vi "IDEGlobals.vi"(6 "task":T1(ring)=enum."write pause", 9 "Port":string, 10 "Last Path":path, 11 "pause?":bool) -> (1 "Port out":string, 2 "Last Path out":path, 3 "pause? out":bool)   [LabVIEW 2022 SP3]
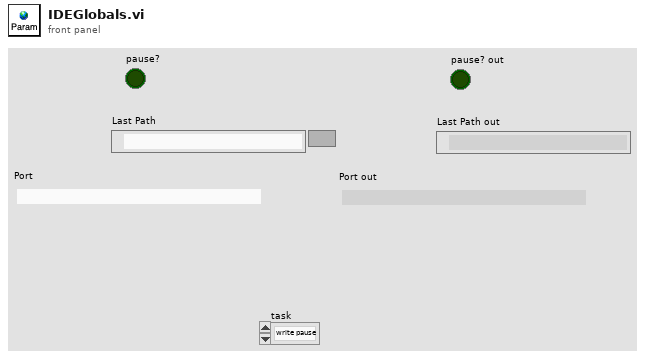
[diagram p1: front panel]
types:
  T1 = enum16{"read", "write pause", "write port", "write path", "write all"}
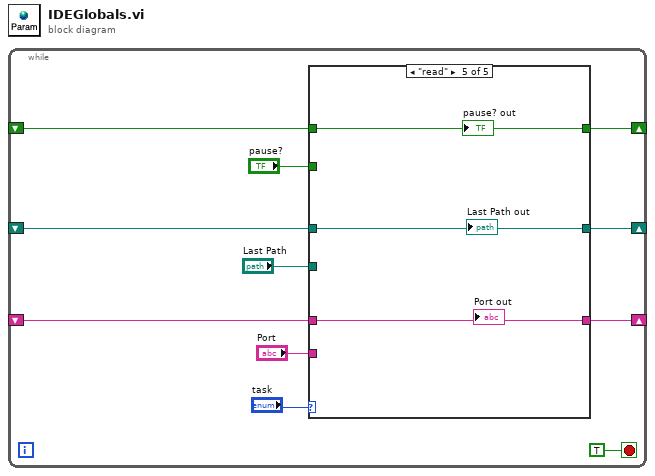
[diagram p0: block diagram]
diagram:
  n1 = while {
    shift-right: [w5] -> _
    shift-left: _ -> [w10]
    shift-right: [w6] -> _
    shift-left: _ -> [w9]
    shift-right: [w7] -> _
    shift-left: _ -> [w8]
    stop <- TRUE stop-if-true
    n2 = case shown="\"read\"" "task" {
      tunnel: w10 -> [_ w16 w19 _ w26]
      tunnel: w9 -> [w13 w15 _ _ w25]
      tunnel: w8 -> [w12 _ w18 _ w24]
      tunnel: [w12 w17 w18 w21 w24] -> w7
      tunnel: [w13 w15 w20 w22 w25] -> w6
      tunnel: [w14 w16 w19 w23 w26] -> w5
      tunnel: "pause?" -> [w14 _ _ w23 _]
      tunnel: "Last Path" -> [_ _ w20 w22 _]
      tunnel: "Port" -> [_ w17 _ w21 _]
      frame "write pause", Default {
      }
      frame "write port" {
      }
      frame "write path" {
      }
      frame "write all" {
      }
      frame "read" {
        "pause? out" <- w26
        "Last Path out" <- w25
        "Port out" <- w24
      }
    }
  }
